vi "Multiple AI Monitor FPGA (Main).vi"() -> ()   [LabVIEW 2010]
panel:
  out "AI2 value":i16
  in  "Maximum Limit (AI2)":i16=32767
  in  "AI2 Scan Period (us)":u32
  out "DIO2":bool
  out "AI1 value":i16
  in  "Maximum Limit (AI1)":i16=32767
  in  "AI1 Scan Period (us)":u32
  out "DIO1":bool
  out "DIO0":bool
  in  "AI0 Scan Period (us)":u32
  out "AI0 value":i16
  in  "Maximum Limit (AI0)":i16=32767
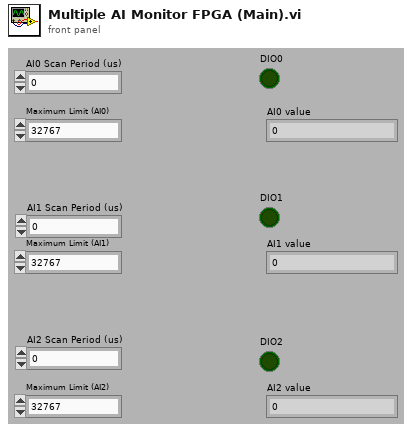
[diagram p1: front panel]
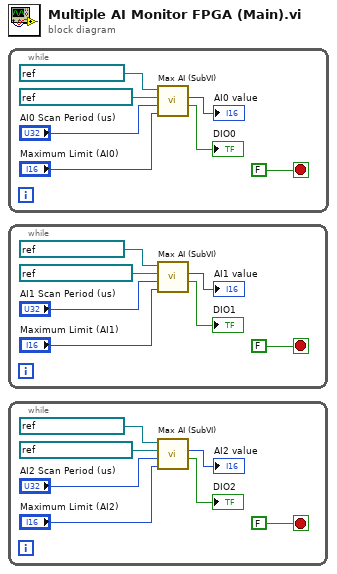
[diagram p0: block diagram]
diagram:
  n1 = while {
    stop <- FALSE stop-if-true
    n2 = call "Max AI (SubVI).vi"("Threshold"="Maximum Limit (AI0)", "AI Scan Period (us)"="AI0 Scan Period (us)", "Digital Output"=refnum<k21> "Connector0/DIO0", "Analog Input"=refnum<k21> "Connector0/AI0") -> ("Threshold Reached"=→"DIO0":bool, "AI value"=→"AI0 value":i16)  [unwired: 6 out]
  }
  n3 = while {
    stop <- FALSE stop-if-true
    n4 = call "Max AI (SubVI).vi"("Threshold"="Maximum Limit (AI1)", "AI Scan Period (us)"="AI1 Scan Period (us)", "Digital Output"=refnum<k21> "Connector0/DIO1", "Analog Input"=refnum<k21> "Connector0/AI1") -> ("Threshold Reached"=→"DIO1":bool, "AI value"=→"AI1 value":i16)  [unwired: 6 out]
  }
  n5 = while {
    stop <- FALSE stop-if-true
    n6 = call "Max AI (SubVI).vi"("Threshold"="Maximum Limit (AI2)", "AI Scan Period (us)"="AI2 Scan Period (us)", "Digital Output"=refnum<k21> "Connector0/DIO2", "Analog Input"=refnum<k21> "Connector0/AI2") -> ("Threshold Reached"=→"DIO2":bool, "AI value"=→"AI2 value":i16)  [unwired: 6 out]
  }
